vi "web-service.vi"() -> ()   [LabVIEW 2014]
panel:
  in  "Cancel":bool
  out "Slide":dbl(slide) scale=0.0..100.0
  in  "Knob":dbl(knob) scale=0.0..100.0
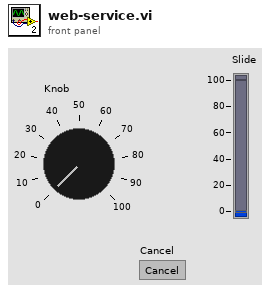
[diagram p1: front panel]
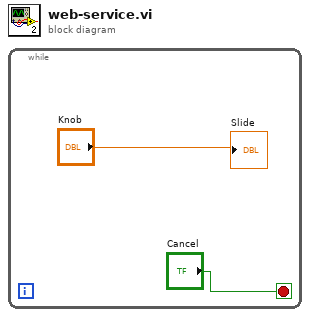
[diagram p0: block diagram]
diagram:
  n1 = while {
    stop <- "Cancel" stop-if-true
    "Slide" <- "Knob"
  }
